vi "Change menu button color as per screen index.vi"(8 "error in (no error)":errorcluster, 10 "Screen Index":i32, 11 "Array":refnum<vi>[](array[refnum])) -> (0 "error out":errorcluster)   [LabVIEW 2023]
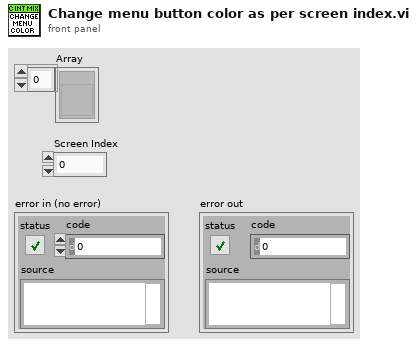
[diagram p1: front panel]
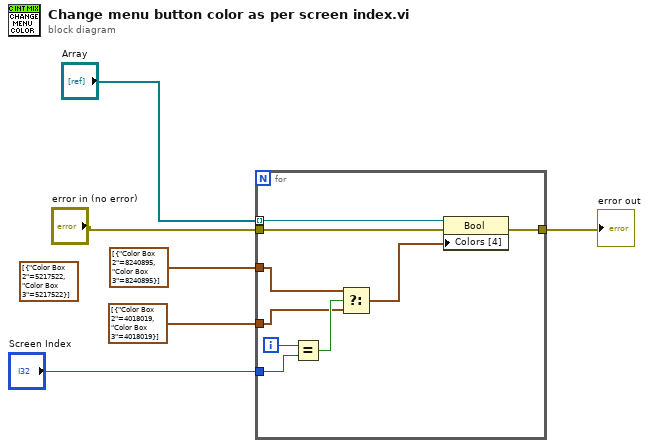
[diagram p0: block diagram]
diagram:
  (unwired) cluster{"Color Box 2":u32, "Color Box 3":u32}[] [{"Color Box 2"=5217522, "Color Box 3"=5217522}] ("Colors [4]")
  n1 = for {
    tunnel: "Array" -> [w10] mode=indexing
    tunnel: cluster{"Color Box 2":u32, "Color Box 3":u32}[] [{"Color Box 2"=8240895, "Color Box 3"=8240895}] ("Colors [4]") -> [w11]
    tunnel: cluster{"Color Box 2":u32, "Color Box 3":u32}[] [{"Color Box 2"=4018019, "Color Box 3"=4018019}] ("Colors [4]") -> [w12]
    tunnel: "Screen Index" -> [w14]
    tunnel: [w8] -> w6
    tunnel: "error in (no error)" -> [w7]
    i -> [w15]
    n2 = Equal?(x=w15, y=w14) -> (x = y?=w13:bool)
    n3 = Select(t=w11, s=w13, f=w12) -> (s? t:f=w9:cluster{"Color Box 2":u32, "Color Box 3":u32}[])
    n4 = property class="Bool"(reference=w10, error in=w7, "Colors [4]"=w9) -> (error out=w8:errorcluster)  [unwired: 1 out]
  }
  "error out" <- w6
